vi "Redirect URI.vi"(11 "Request in":refnum<class "Request.lvclass">) -> (2 "Redirect URI":refnum<class "URI.lvclass">)   [LabVIEW 2020, in "OAuth2.lvlib" / "Request.lvclass"]
uses:
  Request.lvclass
  lv-stream/stream/URI/URI.lvclass
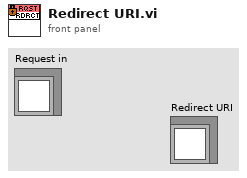
[diagram p1: front panel]
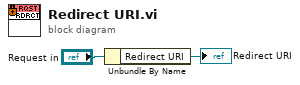
[diagram p0: block diagram]
diagram:
  n1 = Unbundle By Name("Request in") -> ("Redirect URI"=→"Redirect URI":refnum<class "URI.lvclass">)
